vi "medicaoIXV.vi"() -> ()   [LabVIEW 2012]
uses:
  <vilib>/Utility/file.llb/Write To Spreadsheet File (string).vi
  <vilib>/Utility/file.llb/Write To Spreadsheet File (DBL).vi
  <instrlib>/Agilent 6XXX Series/Agilent 6XXX Series.lvlib
panel:
  in  "Tab Control":enum32{"Entrada de dados", "Saída de dados"}(tab)
  out "ON/OFF":bool
  in  "Pontos":dbl
  in  "Tensão máxima":dbl
  in  "Nome da célula":string
  in  "Local":path
  in  "Delay(s)":dbl
  in  "Start":bool
  out "IXV":cluster{"Y":dbl[], "Y":dbl[]}[](graph)
  out "output voltage":dbl
  out "Tensao Atual":dbl
  out "Corrente Atual":dbl
  out "Ponto Atual":i32
  out "TABELA DE DADOS\nTensão(fonte)     Tensão                  Corrente            Pontos":dbl[][](array[numeric]) caption="all rows" format="%0.3f"
  in  "CorrenteGraph":dbl
  in  "error in (no error)":errorcluster
  out "error out":errorcluster
  in  "TensaoGraph":dbl
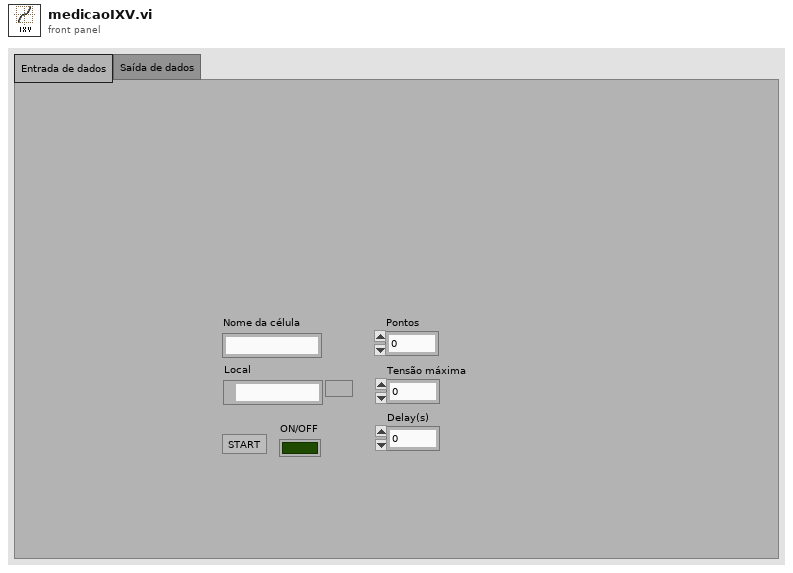
[diagram p1: front panel]
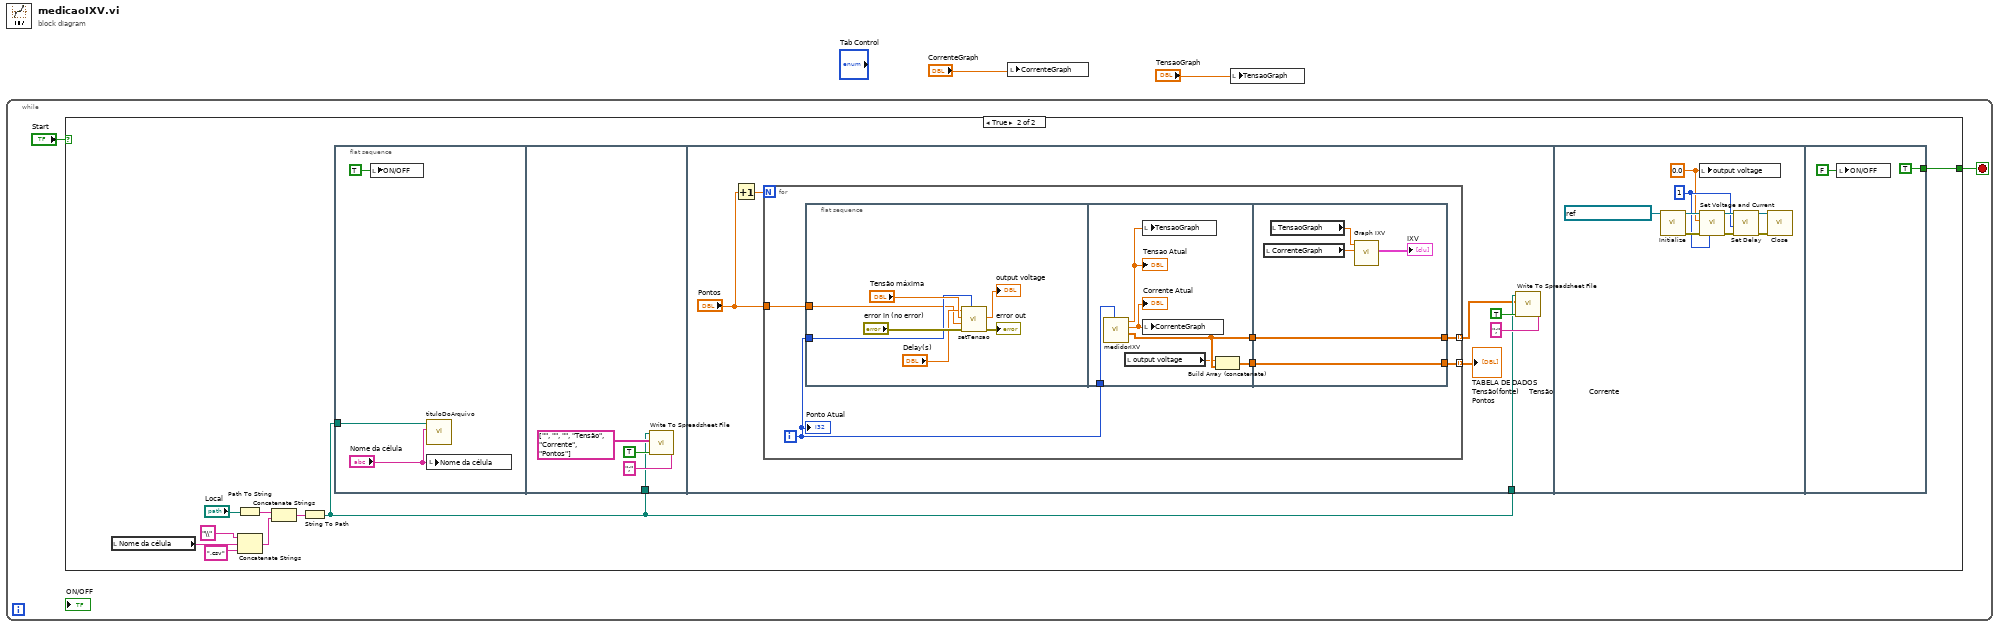
[diagram p0: block diagram]
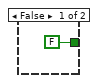
[diagram p2: hidden frame]
diagram:
  n1 = while {
    stop <- w3 stop-if-true
    n2 = case shown="True" "Start" {
      tunnel: [FALSE w8] -> w3
      frame False {
      }
      frame True {
        n3 = local read "Nome da célula"() -> (w9:string)
        n4 = Path To String(path="Local") -> (string=w13:string)
        n5 = Concatenate Strings("\\", w9, ".csv") -> (w14:string)
        n6 = Concatenate Strings(w13, w14) -> (w12:string)
        n7 = String To Path(string=w12) -> (path=w6:path)
        n8 = flat-sequence {
          tunnel: w6 -> [w16]
          tunnel: w6 -> [w18]
          tunnel: w6 -> [w26]
          tunnel: [TRUE] -> w8
          frame #0 {
            n9 = local write "ON/OFF"(TRUE ("ON/OFF")) -> ()
            n10 = call "tituloDoArquivo.vi"("Nome da célula"="Nome da célula", "file path (dialog if empty)"=w16) -> ()  [unwired: 10 in]
            n11 = local write "Nome da célula"("Nome da célula") -> ()
          }
          frame #1 {
            n12 = call-poly <vilib>:"Write To Spreadsheet File.vi"("delimiter (\\t)"=";" ("delimiter (\\t)"), "append to file? (new file:F)"=TRUE, "2D data"=string[][] [["", "", ""], ["Tensão", "Corrente", "Pontos"]], "file path (dialog if empty)"=w18) -> ()  [unwired: 4 in, 1 out]
          }
          frame #2 {
            n13 = Increment(x="Pontos") -> (x+1=w25:dbl)
            n14 = for {
              N: w25 -> [_]
              tunnel: [w32] -> w23 mode=indexing
              tunnel: "Pontos" -> [w34]
              tunnel: [w31] -> w22 mode=indexing
              i -> [w33]
              n15 = flat-sequence {
                tunnel: w34 -> [w37]
                tunnel: w33 -> [w38]
                tunnel: w33 -> [w47]
                tunnel: [w44] -> w30
                tunnel: [w42] -> w29
                tunnel: [w51] -> w31
                tunnel: [w52] -> w32
                tunnel: w30 -> [w52]
                tunnel: w29 -> [w51]
                frame #0 {
                  n16 = call "setTensao.vi"("Ponto"=w38, "error in (no error)"="error in (no error)", "Pontos"=w37, "Tensão máxima"="Tensão máxima", "delay(s)"="Delay(s)") -> ("error out"=→"error out":errorcluster, "output voltage"=→"output voltage":dbl)  [unwired: 5 in]
                }
                frame #1 {
                  n17 = call "medidorIXV.vi"("Ponto"=w47) -> ("Array"=w44:dbl[], "Corrente Atual"=w46:dbl, "Tensao Atual"=w45:dbl)  [unwired: 8 in]
                  "Corrente Atual" <- w46
                  "Tensao Atual" <- w45
                  n18 = local read "output voltage"() -> (w43:dbl)
                  n19 = local write "TensaoGraph"(w45) -> ()
                  n20 = local write "CorrenteGraph"(w46) -> ()
                  n21 = Build Array (concatenate)(w43, w44) -> (w42:dbl[])
                }
                frame #2 {
                  n22 = local read "CorrenteGraph"() -> (w48:dbl)
                  n23 = local read "TensaoGraph"() -> (w49:dbl)
                  n24 = call "Graph IXV"("Y Input"=w48, "X Input"=w49) -> ("XY Graph"=→"IXV":cluster{"Y":dbl[], "Y":dbl[]}[])  [unwired: 3 in, 6 out]
                }
              }
              "Ponto Atual" <- w33
            }
            "TABELA DE DADOS\nTensão(fonte)     Tensão                  Corrente            Pontos" <- w22
            n25 = call-poly <vilib>:"Write To Spreadsheet File.vi"("delimiter (\\t)"=";" ("delimiter (\\t)"), "append to file? (new file:F)"=TRUE, "2D data"=w23, "file path (dialog if empty)"=w26) -> ()  [unwired: 4 in, 1 out]
          }
          frame #3 {
            w53 = 0.0 ("voltage (0 V)")
            w56 = u8 1 ("channel (1)")
            n26 = call <instrlib>:"Initialize.vi"("VISA resource name"=refnum<visa-resource-name> "GPIB0::5::INSTR") -> ("error out"=w58:errorcluster, "VISA resource name out"=w57:refnum<visa-resource-name>)  [unwired: 9 in]
            n27 = local write "output voltage"(w53) -> ()
            n28 = call <instrlib>:"Set Voltage and Current.vi"("channel (1)"=w56, "error in (no error)"=w58, "voltage (0 V)"=w53, "VISA resource name"=w57) -> ("error out"=w59:errorcluster, "VISA resource name out"=w60:refnum<visa-resource-name>)  [unwired: 6 in]
            n29 = call <instrlib>:"Set Delay.vi"("error in (no error)"=w59, "channel (1)"=w56, "VISA resource name"=w60) -> ("error out"=w54:errorcluster, "VISA resource name out"=w55:refnum<visa-resource-name>)  [unwired: 7 in]
            n30 = call <instrlib>:"Close.vi"("error in (no error)"=w54, "VISA resource name"=w55) -> ()  [unwired: 9 in, 1 out]
          }
          frame #4 {
            n31 = local write "ON/OFF"(FALSE) -> ()
          }
        }
      }
    }
  }
  n32 = local write "CorrenteGraph"("CorrenteGraph") -> ()
  n33 = local write "TensaoGraph"("TensaoGraph") -> ()
